vi "Keep Front End Ratio.vi"(10 "H/W":dbl, 11 "NewBnds":T1) -> (3 "Front Panel Window:Panel Bounds":T1)   [LabVIEW 2018, in "Support Library.lvlib"]
uses:
  <vilib>/Utility/miscctls.llb/LVRectTypeDef.ctl
  Support Library.lvlib
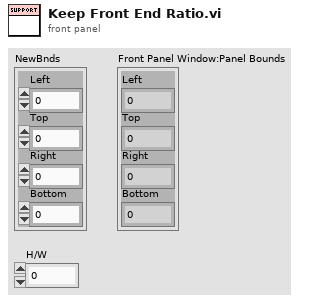
[diagram p1: front panel]
types:
  T1 = typedef "LVRectTypeDef.ctl" = cluster{"Left":i16, "Top":i16, "Right":i16, "Bottom":i16}
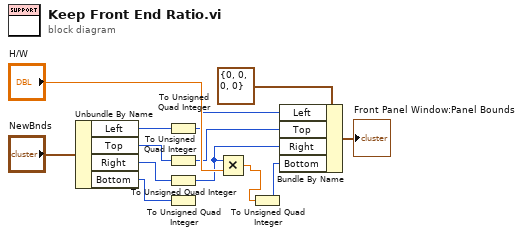
[diagram p0: block diagram]
diagram:
  n1 = Unbundle By Name("NewBnds") -> ("Left"=w11:i16, "Top"=w5:i16, "Right"=w12:i16, "Bottom"=w7:i16)
  n2 = To Unsigned Quad Integer(1:w11) -> (0:w6:u64)
  n3 = To Unsigned Quad Integer(1:w5) -> (0:w4:u64)
  n4 = To Unsigned Quad Integer(1:w12) -> (0:w3:u64)
  n5 = To Unsigned Quad Integer(1:w7) -> ()  [unwired: 1 out]
  n6 = Multiply(x=w3, y="H/W") -> (x*y=w2:dbl)
  n7 = To Unsigned Quad Integer(1:w2) -> (0:w1:u64)
  n8 = Bundle By Name(cluster=T1 {"Left"=0, "Top"=0, "Right"=0, "Bottom"=0} ("Front Panel Window:Panel Bounds"), "Left"=w6, "Top"=w4, "Right"=w3, "Bottom"=w1) -> (→"Front Panel Window:Panel Bounds":T1)
